vi "model.vi"(10 "model inputs":T4, 11 "state in":T1) -> (0 "abort code":i32, 2 "model outputs":T3, 3 "state out":T1)   [LabVIEW 2014, in "Scriptable Model Interface Engine.lvlib"]
uses:
  Scriptable Model Interface Engine.lvlib
  Shared/model outputs.ctl
  Shared/Scriptable Model Interface Shared.lvlib
  Shared/model inputs.ctl
  Shared/model parameters.ctl
  runtime state.ctl
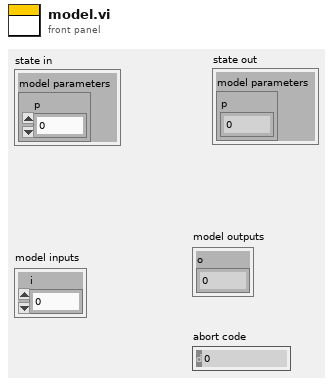
[diagram p1: front panel]
types:
  T1 = typedef "Scriptable Model Interface Engine.lvlib/runtime state.ctl" = cluster{"model parameters":T2}
  T2 = typedef "Scriptable Model Interface Shared.lvlib/model parameters.ctl" = cluster{"p":dbl}
  T3 = typedef "Scriptable Model Interface Shared.lvlib/model outputs.ctl" = cluster{"o":dbl}
  T4 = typedef "Scriptable Model Interface Shared.lvlib/model inputs.ctl" = cluster{"i":dbl}
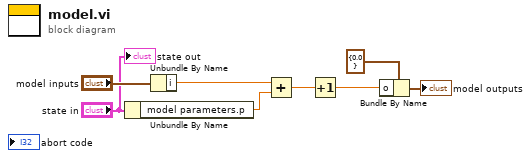
[diagram p0: block diagram]
diagram:
  n1 = Unbundle By Name("state in") -> ("model parameters.p"=w1:dbl)
  n2 = Unbundle By Name("model inputs") -> ("i"=w7:dbl)
  n3 = Add(x=w7, y=w1) -> (x+y=w2:dbl)
  n4 = Increment(x=w2) -> (x+1=w4:dbl)
  n5 = Bundle By Name(cluster=T3 {"o"=0.0} ("model outputs"), "o"=w4) -> (→"model outputs":T3)
  "state out" <- "state in"
